vi "DAQ.TestLauncher.vi"() -> ()   [LabVIEW 2019, in "DAQ.lvclass"]
uses:
  DAQ.lvclass
  <vilib>/JKI/JKI SMO/SMO/SMO.lvclass
  <vilib>/JKI/JKI SMO/SMO/Typedefs/SMOState --Enum.ctl
  C:/Program Files (x86)/National Instruments/LabVIEW 2020/vi.lib/JKI/JKI SMO/SMO/SMO.lvclass
  <vilib>/measure/NI_MABase.lvlib
  Typedefs/DAQ_SamplingMode.ctl
  Typedefs/DAQ_SamplingInfo.ctl
  Typedefs/PrivateEvents--DAQ.AI.Channels.ctl
  Typedefs/DAQ_Type.ctl
  Typedefs/DAQ_Config.ctl
panel:
  in  "AO Waveforms":T1(array[cluster]) {"amplitude" format="%0.2p"; "frequency" format="%0.2p"}
  in  "send new waveform":bool
  out "WRITE event":bool
  out "READ event":bool
  out "WRITE":waveform(dbl)[](graph)
  out "READ":waveform(dbl)[](graph)
  out "SMO Name":string caption="Name"
  in  "DAQ.Config":T2={"Channels"="PXI1Slot2/ao0", "DAQ_Type"=enum."AO", "minimum value"=-5.0, "maximum value"=5.0, "DAQ_SamplingInfo"={"Fs"=1000.0, "#s"=1000}, "DAQ_SamplingMode"=enum."Continuous"} {"maximum value" format="%0.2f"; "minimum value" format="%0.2f"}
  out "SMO State":T7
  out "error out":errorcluster
  in  "Stop":bool
  # "Basic DAQ Test Launcher"
  # "For instructions on how to use the JKI State Machine Objects, examples and video tutorials, visit:\nhttp://jki.net/state-machine-objects/\n\nJKI State Machine Objects™\nhttp://jki.net/state-machine-objects/\nCopyright (C) 2005-2015, JKI <info@jki.net>\nALL RIGHTS RESERVED"
  # "AO will output\nwaveform == 0\nuntil told otherwise"
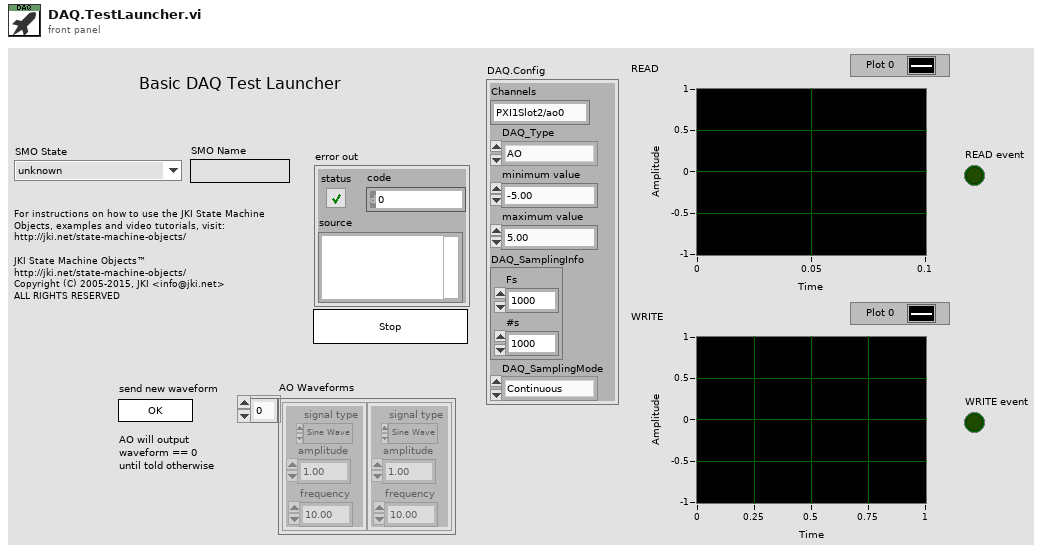
[diagram p1: front panel]
types:
  T1 = cluster{"signal type":enum16{"Sine Wave", "Triangle Wave", "Square Wave", "Sawtooth Wave"}, "frequency":dbl, "amplitude":dbl}[]
  T2 = typedef "DAQ.lvclass/DAQ_Config.ctl" = cluster{"Channels":T3, "DAQ_Type":T4, "minimum value":dbl, "maximum value":dbl, "DAQ_SamplingInfo":T5, "DAQ_SamplingMode":T6}
  T3 = typedef "DAQ.lvclass/PrivateEvents--DAQ.AI.Channels.ctl" = string
  T4 = typedef "DAQ.lvclass/DAQ_Type.ctl" = enum16{"AI", "AO"}
  T5 = typedef "DAQ.lvclass/DAQ_SamplingInfo.ctl" = cluster{"Fs":dbl, "#s":i32}
  T6 = typedef "DAQ.lvclass/DAQ_SamplingMode.ctl" = enum16{"Continuous", "Finite"}
  T7 = typedef "SMO.lvclass/SMOState --Enum.ctl" = enum16{"unknown", "Created", "Started", "Stopped"}
  T8 = typedef "SMO.lvclass/Public Events.ctl" = cluster{"Error":refnum<user-event>, "State":refnum<user-event>, "Reserve State":refnum<user-event>}
  T9 = typedef "DAQ.lvclass/PublicEvents--Cluster.ctl" = cluster{"DAQ.Read":refnum<user-event>, "DAQ.Write":refnum<user-event>}
  T10 = cluster{"Event Registration Refnum":refnum<event-registration>}
  T11 = enum16{"Sine Wave", "Triangle Wave", "Square Wave", "Sawtooth Wave"}
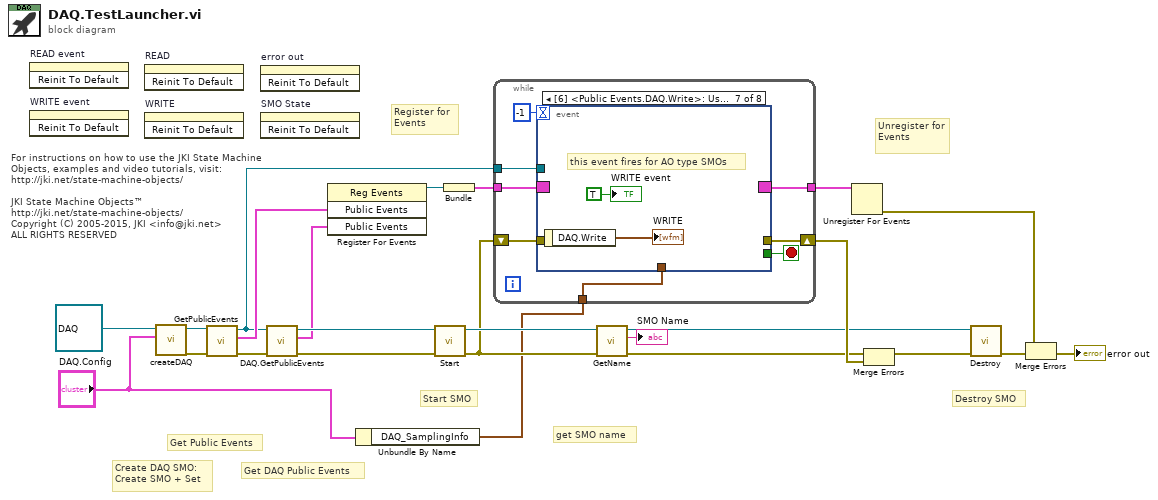
[diagram p0: block diagram]
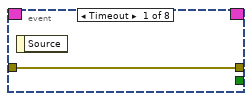
[diagram p2: hidden frame]
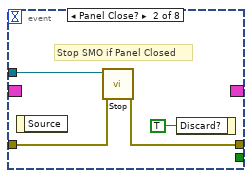
[diagram p3: hidden frame]
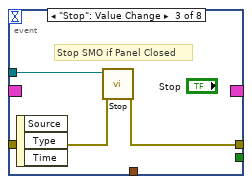
[diagram p4: hidden frame]
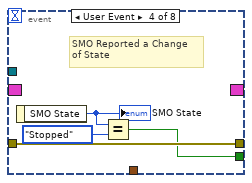
[diagram p5: hidden frame]
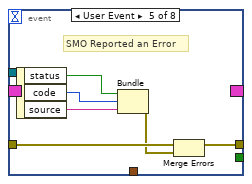
[diagram p6: hidden frame]
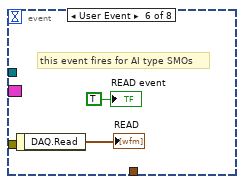
[diagram p7: hidden frame]
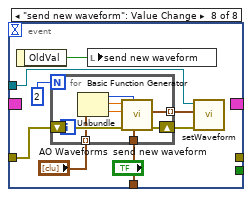
[diagram p8: hidden frame]
diagram:
  # "get SMO name"
  # "Get DAQ Public Events"
  # "For instructions on how to use the JKI State Machine Objects, examples and video tutorials, visit:\nhttp://jki.net/state-machine-objects/\n\nJKI State Machine Objects™\nhttp://jki.net/state-machine-objects/\nCopyright (C) 2005-2015, JKI <info@jki.net>\nALL RIGHTS RESERVED"
  # "Get Public Events"
  # "Start SMO"
  # "Destroy SMO"
  # "Create DAQ SMO:\nCreate SMO + Set"
  # "Unregister for Events"
  # "Register for Events"
  n1 = invoke on="READ event" class="Bool (strict)" method="Reinit To Default"() -> ()  [unwired: 3 in, 3 out]
  n2 = invoke on="WRITE event" class="Bool (strict)" method="Reinit To Default"() -> ()  [unwired: 3 in, 3 out]
  n3 = invoke on="READ" class="WFGraph (strict)" method="Reinit To Default"() -> ()  [unwired: 3 in, 3 out]
  n4 = invoke on="WRITE" class="WFGraph (strict)" method="Reinit To Default"() -> ()  [unwired: 3 in, 3 out]
  n5 = call "createDAQ.vi"("DAQ.Config"="DAQ.Config", "DAQ in"=refnum<class "DAQ.lvclass"> refnum ("SMO.Template.lvclass")) -> ("error out"=w15:errorcluster, "DAQ out"=w13:refnum<class "DAQ.lvclass">)  [unwired: 8 in]
  n6 = call <vilib>:"GetPublicEvents.vi"("error in (no error)"=w15, "SMO"=w13) -> ("error out"=w7:errorcluster, "Public Events"=w17:T8, "SMO out"=w6:refnum<class "DAQ.lvclass">)  [unwired: 7 in]
  n7 = invoke on="error out" class="Clust (strict)" method="Reinit To Default"() -> ()  [unwired: 3 in, 3 out]
  n8 = invoke on="SMO State" class="Enum (strict)" method="Reinit To Default"() -> ()  [unwired: 3 in, 3 out]
  n9 = call "DAQ.GetPublicEvents.vi"("error in (no error)"=w7, "DAQ"=w6) -> ("error out"=w4:errorcluster, "Public Events"=w3:T9, "DAQ out"=w5:refnum<class "DAQ.lvclass">)  [unwired: 7 in]
  n10 = register-events(w17, w3) -> (reference out=w16:refnum<event-registration>)  [unwired: 2 in, 1 out]
  n11 = Unbundle By Name("DAQ.Config") -> ("DAQ_SamplingInfo"=w1:T5)
  n12 = call <vilib>:"Start.vi"("error in (no error)"=w4, "SMO"=w5) -> ("error out"=w9:errorcluster, "SMO out"=w11:refnum<class "DAQ.lvclass">)  [unwired: 8 in]
  n13 = Bundle("Event Registration Refnum"=w16) -> (w23:T10)  [unwired: 1 in]
  n14 = while {
    shift-right: [w31] -> w22
    shift-left: w9 -> [w30]
    tunnel: w23 -> [w29]
    tunnel: [w28] -> w24
    tunnel: w6 -> [w27]
    tunnel: w1 -> [w25]
    stop <- w32 stop-if-true
    n15 = event shown="[6] <Public Events.DAQ.Write>: User Event" {
      selector: w29 -> [_ _ _ _ _ _ _ _]
      dyn-events: [_ _ _ _ _ _ _ _] -> w28
      timeout: -1 -> [_ _ _ _ _ _ _ _]
      tunnel: [_ _ _ w41 _ _ _ _] -> w32
      tunnel: w27 -> [_ w37 w40 _ _ _ _ w58]
      tunnel: [w33 w36 w39 w44 w48 _ _ _] -> w31
      tunnel: w30 -> [w33 w35 w38 w44 w46 _ _ w60]
      tunnel: w25 -> [_ _ _ _ _ _ _ w56]
      event Timeout {
        n16 = event-data() -> ()  [unwired: 1 in, 1 out]
      }
      event Panel Close? {
        # "Stop SMO if Panel Closed"
        n17 = event-data() -> ()  [unwired: 1 in, 1 out]
        n18 = call <vilib>:"Stop.vi"("error in (no error)"=w35, "SMO"=w37) -> ("error out"=w36:errorcluster)  [unwired: 8 in, 1 out]
        n19 = event-data("Discard?"=TRUE ("OK")) -> ()  [unwired: 1 in, 1 out]
      }
      event "Stop": Value Change {
        # "Stop SMO if Panel Closed"
        n20 = event-data() -> ()  [unwired: 1 in, 3 out]
        n21 = call <vilib>:"Stop.vi"("error in (no error)"=w38, "SMO"=w40) -> ("error out"=w39:errorcluster)  [unwired: 8 in, 1 out]
      }
      event User Event {
        # "SMO Reported a Change\nof State"
        n22 = event-data() -> ("SMO State"=w43:T7)  [unwired: 1 in]
        "SMO State" <- w43
        n23 = Equal?(x=w43, y=SMOState_--Enum."Stopped") -> (x = y?=w41:bool)
      }
      event User Event {
        # "SMO Reported an Error"
        n24 = event-data() -> ("status"=w47:bool, "code"=w50:i32, "source"=w49:string)  [unwired: 1 in]
        n25 = Bundle("status"=w47, "code"=w50, "source"=w49) -> (w45:errorcluster)  [unwired: 1 in]
        n26 = Merge Errors(w46, w45) -> (w48:errorcluster)
      }
      event User Event {
        # "this event fires for AI type SMOs"
        n27 = event-data() -> ("DAQ.Read"=→"READ":waveform(dbl)[])  [unwired: 1 in]
        "READ event" <- TRUE ("READ event")
      }
      event User Event {
        # "this event fires for AO type SMOs"
        n28 = event-data() -> ("DAQ.Write"=→"WRITE":waveform(dbl)[])  [unwired: 1 in]
        "WRITE event" <- TRUE ("WRITE event")
      }
      event "send new waveform": Value Change {
        n29 = event-data() -> ("OldVal"=w55:bool)  [unwired: 1 in]
        n30 = for {
          N: 2 -> [_]
          tunnel: [w70] -> w62 mode=indexing
          shift-right: [w69] -> w61
          shift-left: w60 -> [w68]
          tunnel: "AO Waveforms" -> [w67] mode=indexing
          tunnel: w56 -> [w63]
          n31 = Unbundle(w67) -> ("signal type"=w64:T11, "frequency"=w65:dbl, "amplitude"=w66:dbl)
          n32 = call <vilib>:"Basic Function Generator.vi"("sampling info"=w63, "signal type"=w64, "error in (no error)"=w68, "amplitude"=w66, "frequency"=w65) -> ("error out"=w69:errorcluster, "signal out"=w70:waveform(dbl))  [unwired: 4 in, 1 out]
        }
        n33 = local write "send new waveform"(w55) -> ()
        n34 = call "setWaveform.vi"("error in (no error)"=w61, "setWaveform"=w62, "DAQ"=w58) -> ()  [unwired: 7 in, 2 out]
      }
    }
  }
  n35 = call <vilib>:"GetName.vi"("error in (no error)"=w9, "SMO"=w11) -> ("error out"=w8:errorcluster, "Name"=→"SMO Name":string, "SMO out"=w10:refnum<class "DAQ.lvclass">)  [unwired: 7 in]
  n36 = Unregister For Events(event registration refnum=w24) -> (error out=w21:errorcluster)  [unwired: 1 in]
  n37 = Merge Errors(w8, w22) -> (w18:errorcluster)
  n38 = call <vilib>:"Destroy.vi"("error in (no error)"=w18, "SMO"=w10) -> ("error out"=w19:errorcluster)  [unwired: 9 in]
  n39 = Merge Errors(w21, w19) -> (→"error out":errorcluster)
